vi "transfer_and_submit_job.vi"(8 "error in (no error)":errorcluster, 9 "Password":string, 10 "Username@della.princeton.edu":string, 11 "Experiment Folder":string) -> (0 "error out":errorcluster)   [LabVIEW 2019]
uses:
  ParametersGlobal.vi
panel:
  out "standard error":string
  out "standard output":string
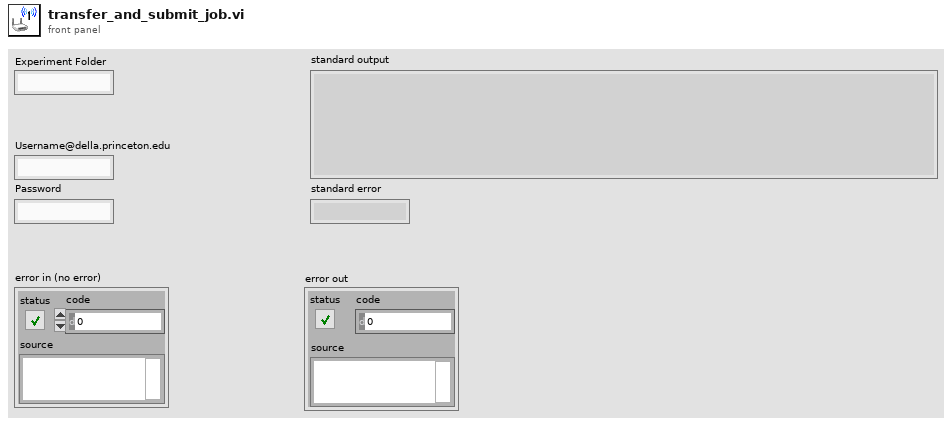
[diagram p1: front panel]
types:
  T1 = enum16{"open", "replace", "create", "open or create", "replace or create", "replace or create with confirmation"}
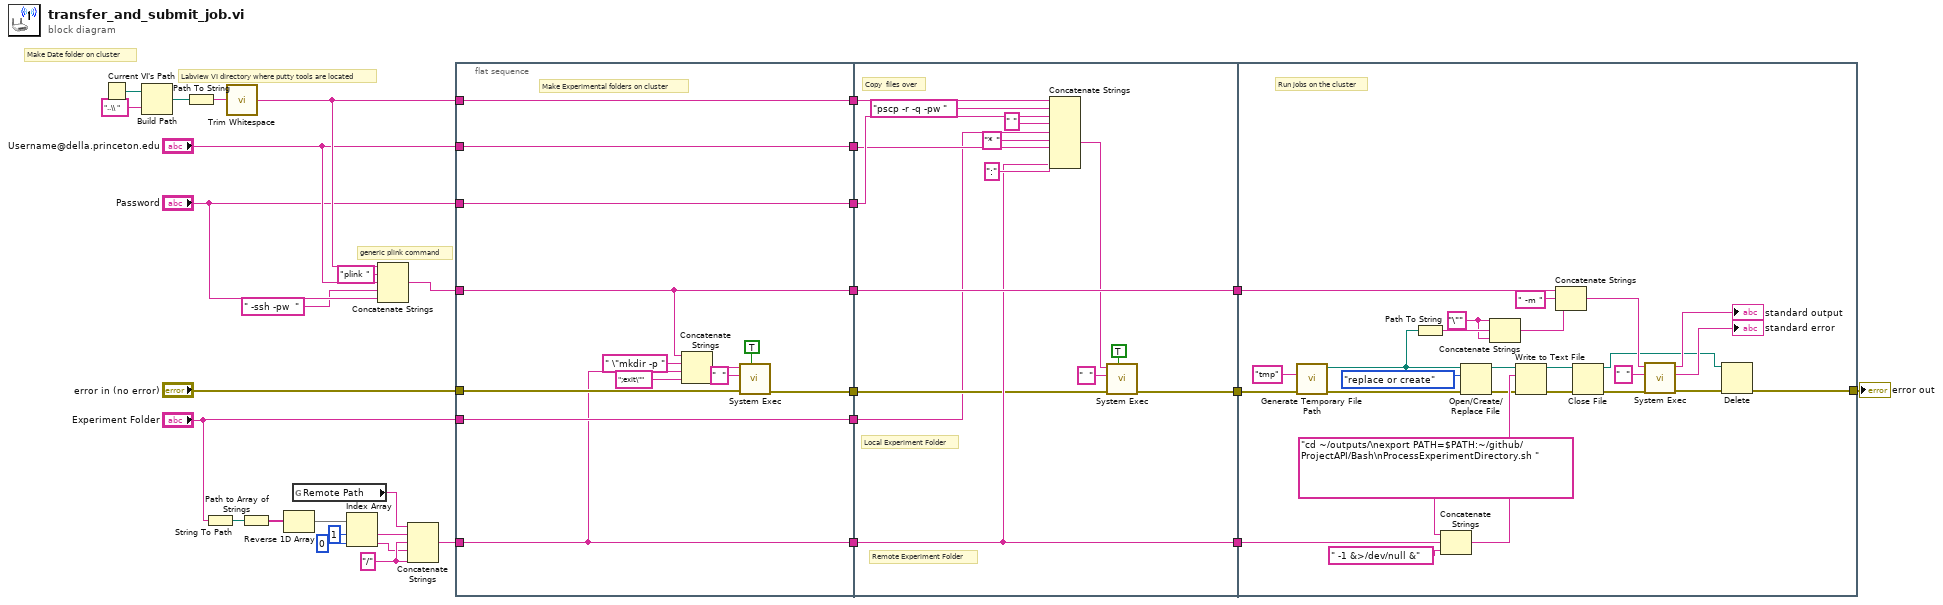
[diagram p0: block diagram]
diagram:
  w5 = "/"
  # "generic plink command"
  # "Make Date folder on cluster"
  # "Labview VI directory where putty tools are located"
  n1 = Current VI's Path() -> (path=w15:path)
  n2 = Build Path(base path=w15, name or relative path="..\\ ") -> (appended path=w17:path)
  n3 = Path To String(path=w17) -> (string=w18:string)
  n4 = String To Path(string="Experiment Folder") -> (path=w11:path)
  n5 = call <vilib>:"Trim Whitespace.vi"("string"=w18) -> ("trimmed string"=w22:string)  [unwired: 1 in]
  n6 = Path to Array of Strings(0:w11) -> (2:w8:string[])  [unwired: 1 out]
  n7 = Reverse 1D Array(array=w8) -> (reversed array=w7:string[])
  n8 = global read "ParametersGlobal.vi" "Remote Path"() -> (w12:string)
  n9 = Index Array(array=w7, index #1=1 ("index"), index #2=0 ("index")) -> (element #1=w2:string, element #2=w1:string)
  n10 = Concatenate Strings(w22, "plink ", "Username@della.princeton.edu", " -ssh -pw  ", "Password") -> (w19:string)
  n11 = Concatenate Strings(w12, w2, w5, w1, w5) -> (w6:string)
  n12 = flat-sequence {
    tunnel: [w39] -> w31
    tunnel: [w38] -> w30
    tunnel: [w45] -> w29
    tunnel: w22 -> [w45]
    tunnel: [w34] -> w28
    tunnel: [w37] -> w27
    tunnel: [w40] -> w26
    tunnel: "Username@della.princeton.edu" -> [w39]
    tunnel: "Password" -> [w38]
    tunnel: w19 -> [w37]
    tunnel: "error in (no error)" -> [w36]
    tunnel: "Experiment Folder" -> [w35]
    tunnel: [w35] -> w9
    tunnel: w6 -> [w34]
    tunnel: w31 -> [w55]
    tunnel: w30 -> [w58]
    tunnel: w29 -> [w59]
    tunnel: [w53] -> w25
    tunnel: w28 -> [w53]
    tunnel: [w61] -> w24
    tunnel: w27 -> [w61]
    tunnel: w26 -> [w49]
    tunnel: [w48] -> w23
    tunnel: w9 -> [w47]
    tunnel: w25 -> [w68]
    tunnel: w24 -> [w67]
    tunnel: w23 -> [w66]
    tunnel: [w63] -> w32
    frame #0 {
      # "Make Experimental folders on cluster"
      n13 = Concatenate Strings(w37, " \"mkdir -p ", w34, ";exit\"") -> (w41:string)
      n14 = call <vilib>:"System Exec.vi"("wait until completion? (T)"=TRUE, "error in (no error)"=w36, "standard input"="  ", "command line"=w41) -> ("error out"=w40:errorcluster)  [unwired: 4 in, 3 out]
    }
    frame #1 {
      # "Remote Experiment Folder"
      # "Local Experiment Folder"
      # "Copy  files over"
      n15 = Concatenate Strings(w59, "pscp -r -q -pw ", w58, " ", w47, "* ", w55, ":", w53) -> (w50:string)
      n16 = call <vilib>:"System Exec.vi"("wait until completion? (T)"=TRUE, "error in (no error)"=w49, "standard input"="  ", "command line"=w50) -> ("error out"=w48:errorcluster)  [unwired: 4 in, 3 out]
    }
    frame #2 {
      w64 = "\""
      # "Run jobs on the cluster"
      n17 = call <vilib>:"Generate Temporary File Path.vi"("error in (no error)"=w66, "Temporary File Extension (tmp)"="tmp") -> ("error out"=w74:errorcluster, "Unique Temporary File Path"=w80:path)  [unwired: 8 in]
      n18 = Path To String(path=w80) -> (string=w65:string)
      n19 = Concatenate Strings("cd ~/outputs/\nexport PATH=$PATH:~/github/ProjectAPI/Bash\nProcessExperimentDirectory.sh ", w68, " -1 &>/dev/null &") -> (w81:string)
      n20 = Open/Create/Replace File(file path (use dialog)=w80, error in=w74, operation (0:open)=T1."replace or create") -> (refnum out=w75:refnum<file>, error out=w72:errorcluster)  [unwired: 3 in, 1 out]
      n21 = Concatenate Strings(w64, w65, w64) -> (w71:string)
      n22 = Write to Text File(file (use dialog)=w75, text=w81, error in=w72) -> (refnum out=w76:refnum<file>, error out=w73:errorcluster)  [unwired: 1 in, 1 out]
      n23 = Concatenate Strings(w67, " -m ", w71) -> (w82:string)
      n24 = Close File(refnum=w76, error in=w73) -> (error out=w77:errorcluster)  [unwired: 1 out]
      n25 = call <vilib>:"System Exec.vi"("error in (no error)"=w77, "standard input"="  ", "command line"=w82) -> ("error out"=w78:errorcluster, "standard error"=→"standard error":string, "standard output"=→"standard output":string)  [unwired: 5 in, 1 out]
      n26 = Delete(path (use dialog)=w80, error in=w78) -> (error out=w63:errorcluster)  [unwired: 3 in, 2 out]
    }
  }
  "error out" <- w32
